vi "DAQ_TRTD Meas Close.vi"(0 "DAQmx Task In":refnum<k21>, 11 "error in":errorcluster) -> (15 "error out":errorcluster)   [LabVIEW 2021, in "DAQ_Temperature RTD Measurement.lvlib"]
doc: "Aborts and clears the temperature RTD input task"
uses:
  DAQ_Temperature RTD Measurement.lvlib
panel:
  # "Inputs"
  # "Outputs"
  # "Overview:\nThis VI closes the Temperature RTD Measurement task\n\nHardware Requirement:: NI C Series/cDAQ Temperature Input Module (Ex: NI-9217)\n\nSoftware Requirement: NI DAQmx 2022 Q4 or later\n\n\nInstructions:\n1. Input the Temperature RTD Measurement task through DAQmx Task In control\n2. This VI aborts and clears the DAQmx Task"
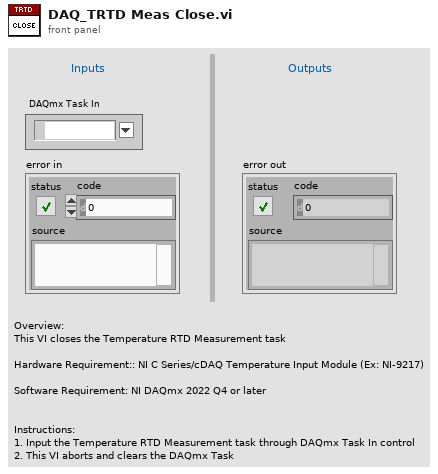
[diagram p1: front panel]
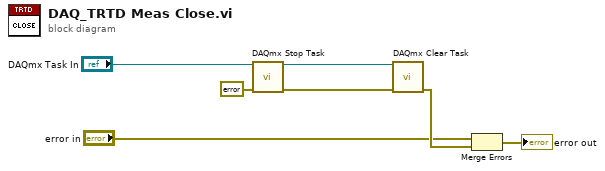
[diagram p0: block diagram]
diagram:
  n1 = call <vilib>:"DAQmx Stop Task.vi"("task/channels in"="DAQmx Task In", "error in"=errorcluster {"status"=FALSE, "code"=0, "source"=""}) -> ("task out"=w6:refnum<k21>, "error out"=w5:errorcluster)  [unwired: 12 in]
  n2 = call <vilib>:"DAQmx Clear Task.vi"("task in"=w6, "error in"=w5) -> ("error out"=w3:errorcluster)  [unwired: 13 in]
  n3 = Merge Errors("error in", w3) -> (→"error out":errorcluster)
